vi "Put PV Data.vi"(7 "PV name":string, 8 "error in":errorcluster, 9 "timeout":dbl[unit]=1.0, 10 "PV Data in":refnum<class "PV Data.lvclass">, 11 "Client in":refnum<class "Client.lvclass">) -> (0 "error out":errorcluster, 1 "timed out?":bool, 3 "Client out":refnum<class "Client.lvclass">)   [LabVIEW 2020, in "PV Access.lvlib" / "PVA Client.lvlib" / "Client.lvclass"]
uses:
  Client.lvclass
  PV Data/PV Data/PV Data.lvclass
  PV Access.lvlib
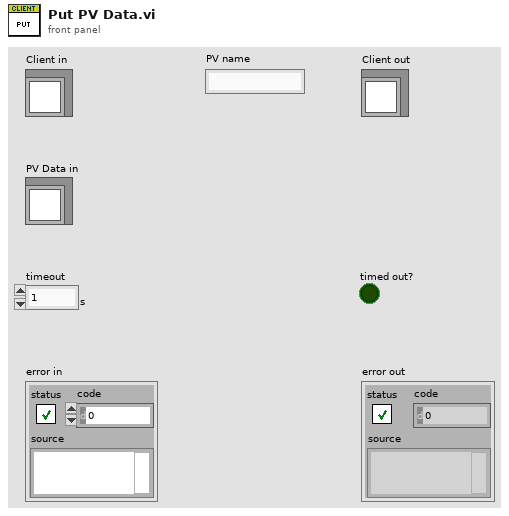
[diagram p1: front panel]
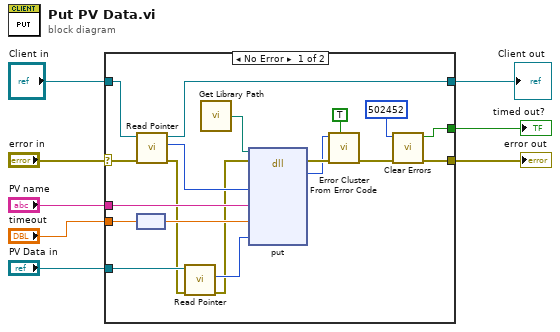
[diagram p0: block diagram]
diagram:
  n1 = case shown="No Error" "error in" {
    selector: "error in" -> [w27 w29]
    tunnel: [w11 w29] -> w5
    tunnel: [w23 w28] -> w4
    tunnel: "Client in" -> [w24 w28]
    tunnel: "PV name" -> [w25 _]
    tunnel: "timeout" -> [w20 _]
    tunnel: "PV Data in" -> [w15 _]
    tunnel: [w9 _] -> w1
    frame No Error {
      n2 = call-dynamic "Read Pointer.vi"("error in (no error)"=w27, "Pointer Base in"=w24) -> ("error out"=w14:errorcluster, "Pointer"=w26:i64, "Pointer Base out"=w23:refnum<class "Client.lvclass">)  [unwired: 7 in]
      n3 = node(w20) -> (w21:dbl)
      n4 = call-dynamic "Read Pointer.vi"("error in (no error)"=w14, "Pointer Base in"=w15) -> ("error out"=w13:errorcluster, "Pointer"=w16:i64)  [unwired: 7 in, 1 out]
      n5 = call "Get Library Path.vi"() -> ("Path"=w22:path)  [unwired: 1 in]
      n6 = dll-call lib="?" fn="put"(path in=w22, error in=w13, "client"=w26, "pv_name"=w25, "timeout"=w21, "value"=w16) -> (error out=w18:errorcluster, "ret_code"=w17:i32)  [unwired: 5 in, 1 out]
      n7 = call <vilib>:"Error Cluster From Error Code.vi"("show call chain? (False)"=TRUE, "error in (no error)"=w18, "error code (0)"=w17) -> ("error out"=w10:errorcluster)  [unwired: 6 in]
      n8 = call <vilib>:"Clear Errors.vi"("error in (no error)"=w10, "specific error code to clear (0: all)"=502452) -> ("error out"=w11:errorcluster, "specific error cleared?"=w9:bool)  [unwired: 4 in]
    }
    frame Error {
    }
  }
  "error out" <- w5
  "Client out" <- w4
  "timed out?" <- w1
